vi "相邻的数组元素相加.vi"(3 "数组输入":u16[](array[numeric])) -> (0 "数组输出":i32[](array[numeric]), 1 "分数":ext)   [LabVIEW 8.6]
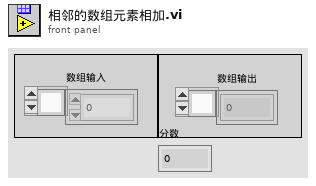
[diagram p1: front panel]
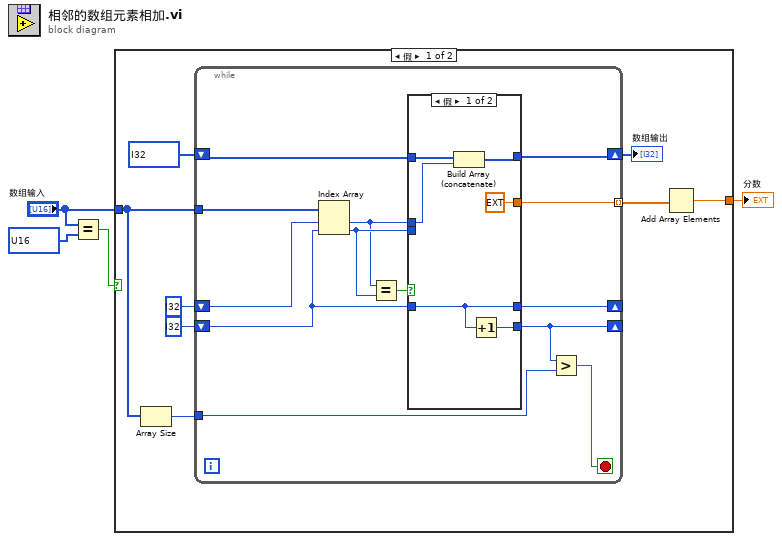
[diagram p0: block diagram]
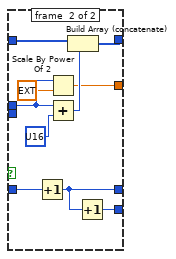
[diagram p2: hidden frame]
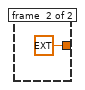
[diagram p3: hidden frame]
diagram:
  n1 = Equal?(x="数组输入", y=u16[] ?) -> (x = y?=w2:bool)
  n2 = case shown="假" w2 {
    tunnel: "数组输入" -> [w7 _]
    tunnel: [w5 ext ?] -> w1
    frame #0 {
      n3 = Array Size(array=w7) -> (size(s)=w9:i32)
      n4 = while {
        tunnel: w7 -> [w25]
        shift-right: [w18] -> _
        shift-left: i32 ? -> [w24]
        shift-right: [w16] -> _
        shift-left: i32 ? -> [w17]
        shift-right: [w20] -> w8
        shift-left: i32[] ? -> [w19]
        tunnel: w9 -> [w15]
        tunnel: [w13] -> w6 mode=indexing
        stop <- w14 stop-if-true
        n5 = Index Array(array=w25, index #1=w24, index #2=w17) -> (element #1=w21:u16, element #2=w22:u16)
        n6 = Equal?(x=w21, y=w22) -> (x = y?=w23:bool)
        n7 = case shown="假" w23 {
          tunnel: w22 -> [_ _]
          tunnel: w21 -> [w28 w34]
          tunnel: [w27 w41] -> w20
          tunnel: w19 -> [w29 w40]
          tunnel: [w31 w38] -> w18
          tunnel: w17 -> [w31 w39]
          tunnel: [w30 w37] -> w16
          tunnel: [ext ? w32] -> w13
          frame #0 {
            n8 = Build Array (concatenate)(w29, w28) -> (w27:i32[])
            n9 = Increment(x=w31) -> (x+1=w30:i32)
          }
          frame #1 {
            n10 = Increment(x=w39) -> (x+1=w38:i32)
            n11 = Scale By Power Of 2(n=w34, x=ext ?) -> (x*2^n=w32:ext)
            n12 = Add(x=w34, y=u16 ?) -> (x+y=w35:u16)
            n13 = Build Array (concatenate)(w40, w35) -> (w41:i32[])
            n14 = Increment(x=w38) -> (x+1=w37:i32)
          }
        }
        n15 = Greater?(x=w16, y=w15) -> (0:w14:bool)
      }
      "数组输出" <- w8
      n16 = Add Array Elements(numeric array=w6) -> (sum=w5:ext)
    }
    frame #1 {
    }
  }
  "分数" <- w1
